vi "LVFPGA Tx Cont Optimized.vi"(0 "device name":string="RIO0", 1 "Enabled Channels":string(combo)="0", 5 "IQ rate":dbl=10000000.0 caption="IQ Rate" format="%#.3pS/s", 7 "number of samples":i64=16384 caption="Number of Samples", 9 "run duration":dbl=5.0 format="%#_13g", 11 "error in":errorcluster) -> (6 "coerced IQ rate":dbl format="%#_6p", 8 "underflow":bool, 10 "overflow":bool, 15 "error out":errorcluster)   [LabVIEW 2015]
doc: "This template is for the Simple NI-USRP Streaming design, a design that shows the basics of streaming data to an NI USRP-294x/295x device. Refer to the block diagram for more information about how to use this template."
uses:
  SubVIs/niusrprios Start Trigger.ctl
  SubVIs/niusrprios Streaming Xvcr FPGA Ref.ctl
  SubVIs/niusrprios Configure Signal (Level).vi
  SubVIs/niusrprios Write Tx Data (I16 multi).vi
  <vilib>/Utility/error.llb/Error Cluster From Error Code.vi
  <vilib>/rvi/errors/niLvFpgaAdjustHostInterfaceError.vi
  <vilib>/rvi/interface/nirviMethod/nirviMethod.xnode
  <vilib>/FPGAPlugInAG/Dynamic/niLvFpga_WriteFifo_Dynamic.vi
  <vilib>/rvi/errors/niLvFpgaMergeErrorWithErrorCode.vi
panel:
  out "error out before clear":errorcluster
  in  "which bitfile":string(combo)="Time"
  in  "Reference Frequency Source":string(combo)="Internal"
  out "generating":bool caption="Generating"
  in  "stop":bool
  # "Tx Streaming"
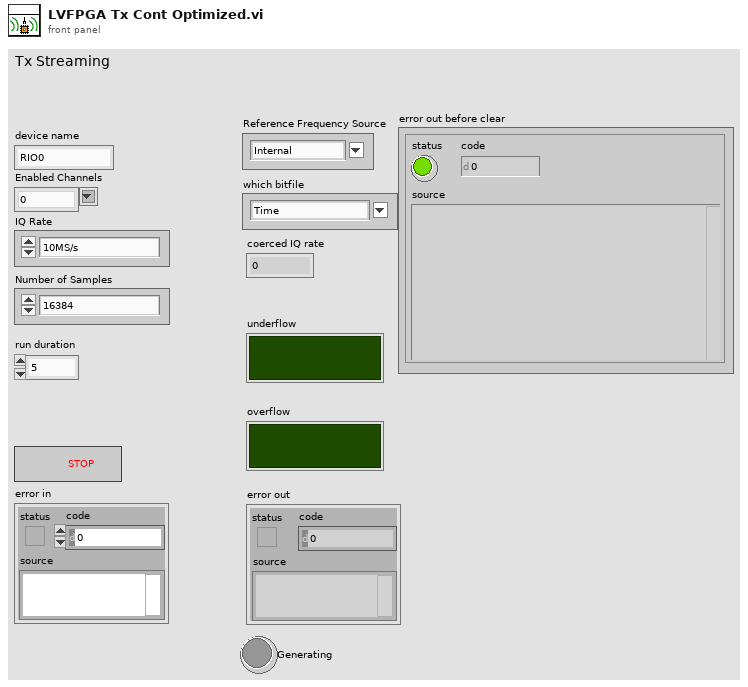
[diagram p1: front panel]
types:
  T1 = typedef "niusrprios Streaming Xvcr FPGA Ref.ctl" = refnum<k20>
  T2 = typedef "niusrprios Start Trigger.ctl" = enum8{"Software", "Digital Edge", "Rx Start Trigger", "Tx Start Trigger", "Immediate", "Future Time Event"}
  T3 = cluster{"antenna":string, "frequency":dbl, "lo frequency":dbl, "level":dbl}
  T4 = cluster{"channel enable":bool, "channel configuration":cluster{"antenna":string, "frequency":dbl, "lo frequency":dbl, "level":dbl}}
  T5 = cluster{"antenna":string, "frequency":dbl, "lo frequency":dbl, "level":dbl}[]
  T6 = typedef "niUsrpRio Config v1 Host.lvlib/niUsrpRio Session.ctl" = cluster{"FPGA Interface":refnum<k20>, "RIO Interface Number":u32, "Data Clock Rate":u32, "FPGA Data Clock Rate":u32, "Global Settings Register Bus":T7, "Radio 0 Settings Register Bus":T7, "Radio 1 Settings Register Bus":T7, "Radio Settings Bus Semaphore":T8, "DB Queues":T9[], "Characterization Data Valid?":bool, "EEPROM Header":T10, "Device Data Header":T11, "EEPROM Characterization Header":T12, "Characterization Data":T13[], "FPGA Current Version":u32, "FPGA Oldest Compatible Version":u32, "Fixed Logic Current Version":u32, "Fixed Logic Oldest Compatible Version":u32, "FPGA Radio Settings Bus Current Version":u32, "FPGA Radio Settings Bus Oldest Compatible Version":u32, "FPGA Board Config Current Version":u32, "FPGA Board Config Oldest Compatible Version":u32, "Daughterboard Clock Rate":u32}
  T7 = typedef "niInstr Register Bus v0 Host.lvlib/Register Bus Session.ctl" = refnum<queue>
  T8 = typedef "Semaphore RefNum" = refnum<k1>
  T9 = typedef "niUsrpRio Config v1 Host.lvlib/DB Queue Reference.ctl" = refnum<queue>
  T10 = typedef "niUsrpRio Config v1 Host.lvlib/EEPROM Header.ctl" = cluster{"Checksum":u32, "Product Code":u16, "Hardware Current Version":u16, "Hardware Oldest Compatible Version":u16, "EEPROM Map Current Version":u16, "EEPROM Map Oldest Compatible Version":u16, "User Password":string, "Pointer to Factory Header":u32, "Pointer to User Header":u32, "Recommended Interval":u16, "Number of Reserved Bytes":i32, "Number of Daughterboards":u8, "Daughterboard IDs":u16[], "Daughterboard Serial Numbers":string[]}
  T11 = typedef "niUsrpRio Config v1 Host.lvlib/EEPROM Device Data Header.ctl" = cluster{"Checksum":u32, "Number of Channels":u8, "Number of Gain Settings":u16[], "Pointer to Characterization Data":u32[], "Number of Reserved Bytes":i32, "Number of Frequencies":u16[]}
  T12 = typedef "niUsrpRio Config v1 Host.lvlib/EEPROM Characterization Header.ctl" = cluster{"Checksum":u32, "Date":timestamp, "Temperature":sgl, "Misc. Info":string, "Pointer to Device Data Header":u32, "Number of Reserved Bytes":i32}
  T13 = typedef "niUsrpRio Config v1 Host.lvlib/Characterization Data.ctl" = cluster{"Gains[dB]":dbl[], "Frequencies [Hz]":dbl[], "IQ Imbalance Table":T14[], "Measured Gains[dB]":dbl[][]}
  T14 = typedef "niUsrpRio Config v1 Host.lvlib/IQ Imbalance.ctl" = cluster{"Gain Imbalance [linear]":dbl, "Phase Imbalance [radians]":dbl, "Offset":cdb}
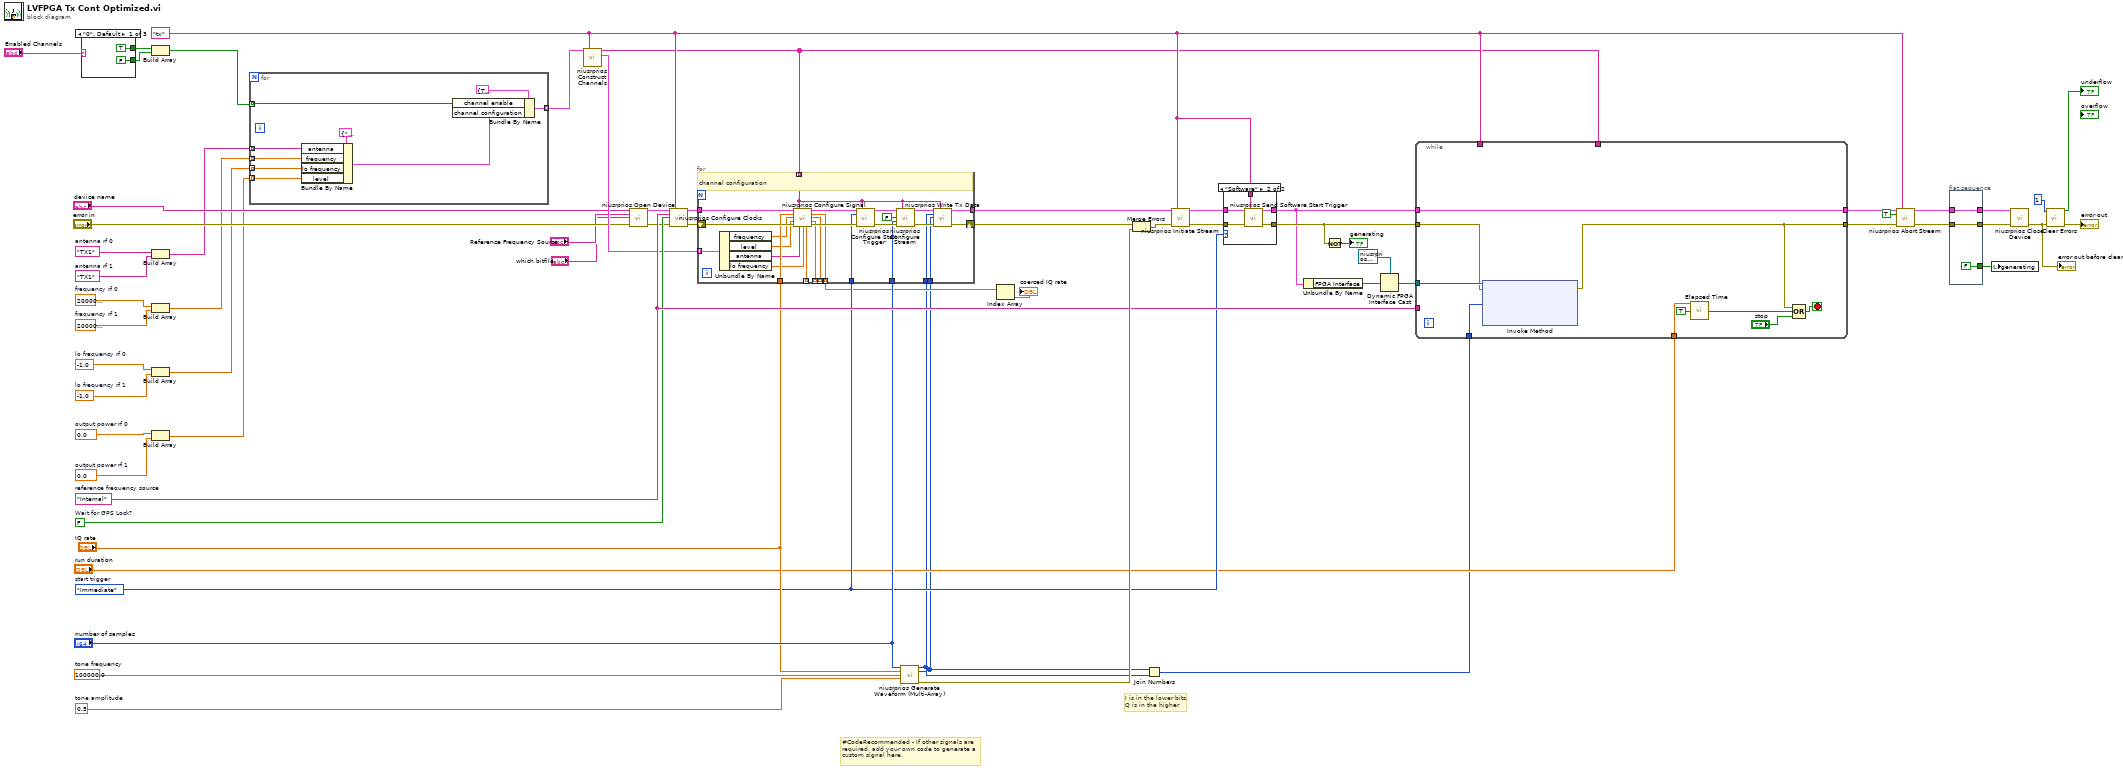
[diagram p0: block diagram]
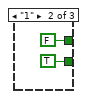
[diagram p2: hidden frame]
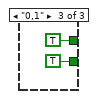
[diagram p3: hidden frame]
diagram:
  w51 = 100000.0  # tone frequency
  w42 = niusrprios_Start_Trigger."Immediate"  # start trigger
  w64 = "Internal"  # reference frequency source
  w55 = 0.0  # output power rf 1
  w54 = 0.0  # output power rf 0
  w56 = -1.0  # lo frequency rf 1
  w57 = -1.0  # lo frequency rf 0
  w58 = 2000000000.0  # frequency rf 1
  w59 = 2000000000.0  # frequency rf 0
  w61 = "TX1"  # antenna rf 1
  w60 = "TX1"  # antenna rf 0
  w43 = FALSE  # Wait for GPS Lock?
  w50 = 0.5  # tone amplitude
  w38 = "tx" ("scope")
  # "I is in the lower bits,\nQ is in the higher"
  # "#CodeRecommended - If other signals are required, add your own code to generate a custom signal here."
  n1 = case shown="\"0\", Default" "Enabled Channels" {
    tunnel: [TRUE FALSE TRUE] -> w25
    tunnel: [FALSE TRUE TRUE] -> w24
    frame "0", Default {
    }
    frame "1" {
    }
    frame "0,1" {
    }
  }
  n2 = Build Array(w25, w24) -> (w16:bool[])
  n3 = Build Array(w60, w61) -> (w15:string[])
  n4 = Build Array(w59, w58) -> (w14:dbl[])
  n5 = Build Array(w57, w56) -> (w13:dbl[])
  n6 = Build Array(w54, w55) -> (w12:dbl[])
  n7 = for {
    tunnel: w16 -> [w79] mode=indexing
    tunnel: w15 -> [w77] mode=indexing
    tunnel: w14 -> [w76] mode=indexing
    tunnel: w13 -> [w75] mode=indexing
    tunnel: w12 -> [w74] mode=indexing
    tunnel: [w72] -> w11 mode=indexing
    n8 = Bundle By Name(cluster=T3 {"antenna"="", "frequency"=0.0, "lo frequency"=0.0, "level"=0.0} ("channel configuration"), "antenna"=w77, "frequency"=w76, "lo frequency"=w75, "level"=w74) -> (w73:T3)
    n9 = Bundle By Name(cluster=T4 {"channel enable"=TRUE, "channel configuration"={"antenna"="RX1", "frequency"=2000000000.0, "lo frequency"=-1.0, "level"=0.0}} ("channel configuration"), "channel enable"=w79, "channel configuration"=w73) -> (w72:T4)
  }
  n10 = call "niusrprios Construct Channels.vi"("channel configurations"=w11, "scope"=w38) -> ("enabled channels"=w37:string[], "enabled channel configurations"=w36:T5)  [unwired: 12 in]
  n11 = call "niusrprios Open Device.vi"("USRP RIO device"="device name", "Reference Frequency Source"="Reference Frequency Source", "which bitfile"="which bitfile", "error in"="error in") -> ("niUsrpRio Session (out)"=w35:T6, "error out"=w34:errorcluster)  [unwired: 10 in]
  n12 = call "niusrprios Configure Clocks.vi"("niUsrpRio Session"=w35, "scope"=w38, "Reference Frequency Source"=w64, "GPSDO Power Enable"=w43, "error in"=w34) -> ("niUsrpRio Session (out)"=w32:T6, "error out"=w33:errorcluster)  [unwired: 9 in]
  n13 = call "niusrprios Generate Waveform (Multi-Array).vi"("number of samples"="number of samples", "sample rate"="IQ rate", "tone frequency"=w51, "amplitude"=w50) -> ("I"=w8:i16[], "Q"=w7:i16[], "error out"=w65:errorcluster)  [unwired: 8 in, 1 out]
  n14 = for {
    tunnel: [w90] -> _ mode=indexing
    tunnel: [w95] -> w31
    tunnel: w42 -> [w104]
    tunnel: "number of samples" -> [w99]
    shift-right: [w97] -> w30
    shift-left: w33 -> [w100]
    tunnel: w37 -> [w94] mode=indexing
    tunnel: "IQ rate" -> [w98]
    tunnel: w7 -> [w93]
    tunnel: w8 -> [w92]
    tunnel: w32 -> [w91]
    tunnel: [w89] -> _ mode=indexing
    tunnel: [w88] -> _ mode=indexing
    tunnel: [w87] -> w28 mode=indexing
    tunnel: w36 -> [w86] mode=indexing
    # "channel configuration"
    n15 = Unbundle By Name(w86) -> ("frequency"=w85:dbl, "level"=w84:dbl, "antenna"=w83:string, "lo frequency"=w82:dbl)
    n16 = call-poly "niusrprios Configure Signal.vi"("niUsrpRio Session"=w91, "scope"=w94, "sample rate [S/s]"=w98, "frequency [Hz]"=w85, "level [dBm]"=w84, "error in"=w100, "Active Antenna"=w83, "LO frequency [Hz]"=w82) -> ("niUsrpRio Session (out)"=w102:T6, "coerced sample rate [S/s]"=w87:dbl, "coerced frequency [Hz]"=w88:dbl, "coerced level [dBm]"=w89:dbl, "coerced LO frequency [Hz]"=w90:dbl, "error out"=w106:errorcluster)  [unwired: 1 in, 1 out]
    n17 = call "niusrprios Configure Start Trigger.vi"("niUsrpRio Session"=w102, "scope"=w94, "start trigger"=w104, "error in"=w106) -> ("niUsrpRio Session (out)"=w101:T6, "error out"=w103:errorcluster)  [unwired: 10 in]
    n18 = call "niusrprios Configure Stream.vi"("niUsrpRio Session"=w101, "scope"=w94, "number of samples is finite"=FALSE, "number of samples"=w99, "error in"=w103) -> ("niUsrpRio Session (out)"=w96:T6, "error out"=w105:errorcluster)  [unwired: 9 in]
    n19 = call-poly "niusrprios Write Tx Data.vi"("niUsrpRio Session"=w96, "scope"=w94, "I"=w92, "Q"=w93, "error in"=w105) -> ("niUsrpRio Session (out)"=w95:T6, "error out"=w97:errorcluster)  [unwired: 9 in]
  }
  n20 = Index Array(array=w28) -> (element=→"coerced IQ rate":dbl)  [unwired: 1 in]
  n21 = Merge Errors(w30, w65) -> (w29:errorcluster)
  n22 = Join Numbers(hi=w7, lo=w8) -> ((hi.lo)=w6:u32[])
  n23 = call "niusrprios Initiate Stream.vi"("niUsrpRio Session"=w31, "scope"=w38, "error in"=w29) -> ("niUsrpRio Session (out)"=w39:T6, "error out"=w40:errorcluster)  [unwired: 11 in]
  n24 = case shown="\"Software\"" w42 {
    tunnel: w40 -> [w108 w113]
    tunnel: [w108 w112] -> w41
    tunnel: w39 -> [w107 w111]
    tunnel: w38 -> [_ w110]
    tunnel: [w107 w109] -> w3
    frame Default {
    }
    frame "Software" {
      n25 = call "niusrprios Send Software Start Trigger.vi"("niUsrpRio Session"=w111, "scope"=w110, "error in"=w113) -> ("niUsrpRio Session (out)"=w109:T6, "error out"=w112:errorcluster)  [unwired: 11 in]
    }
  }
  n26 = Unbundle By Name(w3) -> ("FPGA Interface"=w5:refnum<k20>)
  n27 = Not(x=w41) -> (.not. x?=→"generating":bool)
  n28 = Dynamic FPGA Interface Cast(Session In=T1 refnum ("Type"), Type=w5) -> (Session Out=w2:T1)
  n29 = while {
    tunnel: [w115] -> w63
    tunnel: [w114] -> w62
    tunnel: w37 -> [_]
    tunnel: w6 -> [w117]
    tunnel: w41 -> [w116]
    tunnel: w3 -> [w115]
    tunnel: w38 -> [_]
    tunnel: w64 -> [_]
    tunnel: "run duration" -> [w119]
    tunnel: w2 -> [w118]
    stop <- w123 stop-if-true
    # "Acquire and Fetch a waveform"
    n30 = xnode "Invoke Method"("FPGA VI Reference In"=w118, "error in"=w116, "Data"=w117) -> ("error out"=w114:errorcluster)  [unwired: 1 in, 2 out]
    n31 = call "Elapsed Time"("Time Target (s)"=w119, "Auto Reset"=TRUE) -> ("Time has Elapsed"=w120:bool)  [unwired: 10 in, 7 out]
    n32 = Compound Arithmetic op=OR(w114, w120, "stop") -> (w123:bool)
  }
  n33 = call "niusrprios Abort Stream.vi"("niUsrpRio Session"=w63, "scope"=w38, "check stream status"=TRUE, "error in"=w62) -> ("niUsrpRio Session (out)"=w48:T6, "error out"=w49:errorcluster)  [unwired: 10 in]
  n34 = flat-sequence {
    tunnel: [w126] -> w47
    tunnel: w48 -> [w126]
    tunnel: [w125] -> w46
    tunnel: w49 -> [w125]
    tunnel: [FALSE ("Generating")] -> w45
    frame #0 {
    }
  }
  n35 = local write "generating"(w45) -> ()
  n36 = call "niusrprios Close Device.vi"("niUsrpRio Session"=w47, "error in"=w46) -> ("error out"=w22:errorcluster)  [unwired: 13 in]
  "error out before clear" <- w22
  n37 = call <vilib>:"Clear Errors.vi"("error in (no error)"=w22, "specific error code to clear (0: all)"=1) -> ("error out"=→"error out":errorcluster, "specific error cleared?"=→"underflow":bool)  [unwired: 4 in]
